vi "11.2.3.-Momento Invariante de Hu Central - Upq.vi"(0 "xc":dbl, 5 "yc":dbl, 7 "f":dbl[][](array[numeric]), 9 "X":dbl[][](array[numeric]), 11 "Y":dbl[][](array[numeric])) -> (3 "u00":dbl, 4 "u11":dbl, 6 "u12":dbl, 8 "u02":dbl, 10 "u20":dbl, 13 "u30":dbl, 14 "u03":dbl, 15 "u21":dbl)   [LabVIEW 2020]
panel:
  # "Visión Artificial - Momentos Invariantes de Hu\nDiego Cervantes Rodríguez\ndicer0.com"
  # "Momento central = Upq = sum(sum(((X-xc)^p)*((Y-yc)^q)*f(x,y)))"
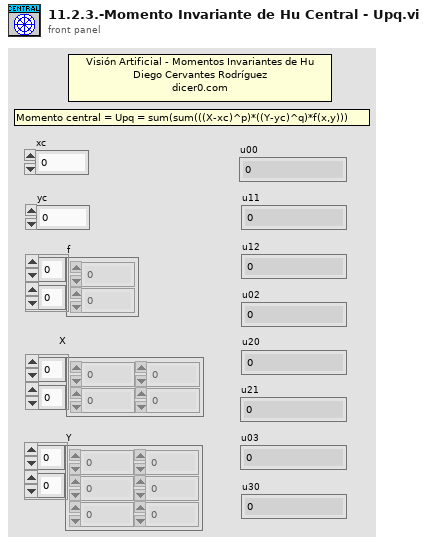
[diagram p1: front panel]
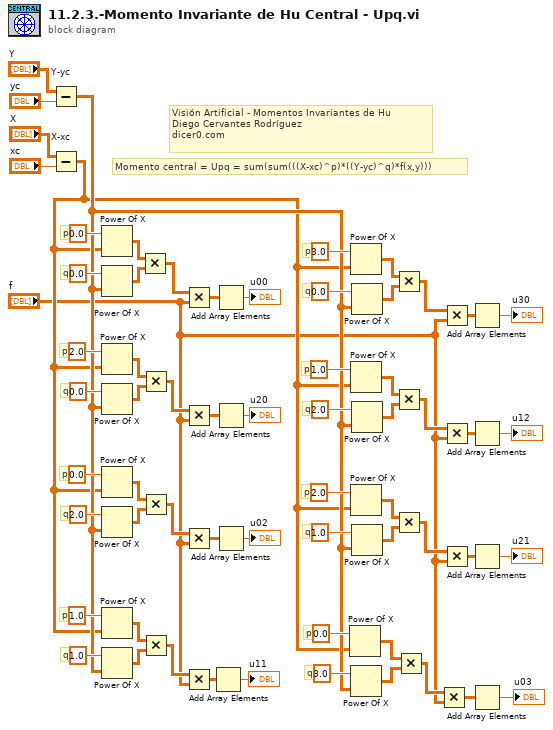
[diagram p0: block diagram]
diagram:
  # "Momento central = Upq = sum(sum(((X-xc)^p)*((Y-yc)^q)*f(x,y)))"
  # "Visión Artificial - Momentos Invariantes de Hu\nDiego Cervantes Rodríguez\ndicer0.com"
  # "q"
  # "p"
  # "p"
  # "q"
  # "p"
  # "q"
  # "q"
  # "p"
  # "q"
  # "p"
  # "p"
  # "q"
  # "p"
  # "q"
  # "q"
  # "p"
  n1 = Subtract "Y-yc"(x="Y", y="yc") -> (x-y=w7:dbl[][])
  n2 = Subtract "X-xc"(x="X", y="xc") -> (x-y=w6:dbl[][])
  n3 = Power Of X(1:w6, 2:0.0) -> (0:w61:dbl[][])
  n4 = Power Of X(1:w7, 2:0.0) -> (0:w60:dbl[][])
  n5 = Power Of X(1:w6, 2:2.0) -> (0:w55:dbl[][])
  n6 = Power Of X(1:w7, 2:0.0) -> (0:w54:dbl[][])
  n7 = Power Of X(1:w6, 2:0.0) -> (0:w49:dbl[][])
  n8 = Power Of X(1:w7, 2:2.0) -> (0:w48:dbl[][])
  n9 = Power Of X(1:w6, 2:1.0) -> (0:w40:dbl[][])
  n10 = Power Of X(1:w7, 2:1.0) -> (0:w39:dbl[][])
  n11 = Multiply(x=w61, y=w60) -> (x*y=w59:dbl[][])
  n12 = Multiply(x=w55, y=w54) -> (x*y=w53:dbl[][])
  n13 = Multiply(x=w49, y=w48) -> (x*y=w47:dbl[][])
  n14 = Multiply(x=w40, y=w39) -> (x*y=w38:dbl[][])
  n15 = Multiply(x=w59, y="f") -> (x*y=w58:dbl[][])
  n16 = Multiply(x=w53, y="f") -> (x*y=w52:dbl[][])
  n17 = Multiply(x=w47, y="f") -> (x*y=w46:dbl[][])
  n18 = Multiply(x=w38, y="f") -> (x*y=w37:dbl[][])
  n19 = Add Array Elements(numeric array=w37) -> (sum=→"u11":dbl)
  n20 = Add Array Elements(numeric array=w58) -> (sum=→"u00":dbl)
  n21 = Add Array Elements(numeric array=w52) -> (sum=→"u20":dbl)
  n22 = Add Array Elements(numeric array=w46) -> (sum=→"u02":dbl)
  n23 = Power Of X(1:w6, 2:0.0) -> (0:w12:dbl[][])
  n24 = Power Of X(1:w6, 2:3.0) -> (0:w33:dbl[][])
  n25 = Power Of X(1:w6, 2:1.0) -> (0:w27:dbl[][])
  n26 = Power Of X(1:w6, 2:2.0) -> (0:w21:dbl[][])
  n27 = Power Of X(1:w7, 2:3.0) -> (0:w11:dbl[][])
  n28 = Power Of X(1:w7, 2:0.0) -> (0:w32:dbl[][])
  n29 = Power Of X(1:w7, 2:2.0) -> (0:w26:dbl[][])
  n30 = Power Of X(1:w7, 2:1.0) -> (0:w20:dbl[][])
  n31 = Multiply(x=w33, y=w32) -> (x*y=w31:dbl[][])
  n32 = Multiply(x=w27, y=w26) -> (x*y=w25:dbl[][])
  n33 = Multiply(x=w21, y=w20) -> (x*y=w19:dbl[][])
  n34 = Multiply(x=w12, y=w11) -> (x*y=w10:dbl[][])
  n35 = Multiply(x=w10, y="f") -> (x*y=w9:dbl[][])
  n36 = Multiply(x=w31, y="f") -> (x*y=w30:dbl[][])
  n37 = Multiply(x=w25, y="f") -> (x*y=w24:dbl[][])
  n38 = Multiply(x=w19, y="f") -> (x*y=w18:dbl[][])
  n39 = Add Array Elements(numeric array=w30) -> (sum=→"u30":dbl)
  n40 = Add Array Elements(numeric array=w24) -> (sum=→"u12":dbl)
  n41 = Add Array Elements(numeric array=w18) -> (sum=→"u21":dbl)
  n42 = Add Array Elements(numeric array=w9) -> (sum=→"u03":dbl)
